vi "CelulaDessalinizadora.vi"() -> ()   [LabVIEW 2014]
panel:
  in  "Adsorção":bool
  in  "OK Button":bool
  in  "Documento de Texto":path
  out "Tempo":dbl
  in  "Condutividade Máxima":dbl
  in  "NÚMERO DE CICLOS":dbl
  in  "Liga/Desliga":bool
  in  "Escolha: Porta Serial":refnum<visa-resource-name>="COM3"
  out "Dessorção":bool
  out "Adsorção":bool
  out "Single-Pass":bool
  out "Batch":bool
  in  "BATCH / SINGLE PASS":bool
  out "Potencial de Célula [mV]":dbl(graph)
  out "pH":dbl(graph)
  out "Condutividade [us/cm]":dbl(graph)
  in  "Selecionar caso":T1(tab)
  in  "TEMPO DE ADSOR敲O P":dbl
  in  "CONDUTIVIDADE \nMÍNIMA NA ADSORÇÃO P":dbl
  in  "TEMPO DE DESSOR敲O P":dbl
  in  "CONDUTIVIDADE \nMÁXIMA NA DESSORÇÃO P":dbl
  in  "Selecionar parâmetro G":enum32{"Tempo", "Condutividade", "Potencial"}(tab)
  in  "TEMPO DE ADSOR敲O G":dbl
  in  "TEMPO DE DESSOR敲O G":dbl
  in  "CONDUTIVIDADE \nMÍNIMA NA ADSORÇÃO G":dbl
  in  "CONDUTIVIDADE \nMÁXIMA NA DESSORÇÃO G":dbl
  in  "POTENCIAL DE CORTE\nNA ADSOR敲O":dbl
  in  "POTENCIAL DE CORTE\nNA DESSOR敲O":dbl
  in  "POTENCIAL DE CORTE\nNA DESSOR敲O G":dbl
  in  "CONDUTIVIDADE \nMÁXIMA NA DESSORÇÃO G2":dbl
  in  "TEMPO DE DESSOR敲O G 2":dbl
  in  "TEMPO DE ADSOR敲O G 2":dbl
  in  "CONDUTIVIDADE \nMÍNIMA NA ADSORÇÃO G 2":dbl
  in  "POTENCIAL DE CORTE\nNA ADSOR敲O G":dbl
  # "CONDUTIVIDADE MÁXIMA"
  # "s"
  # "us/cm"
  # "s"
  # "us/cm"
  # "s"
  # "s"
  # "us/cm"
  # "us/cm"
  # "VV"
  # "V"
  # "s"
  # "us/cm"
  # "mV"
  # "s"
  # "us/cm"
  # "mV"
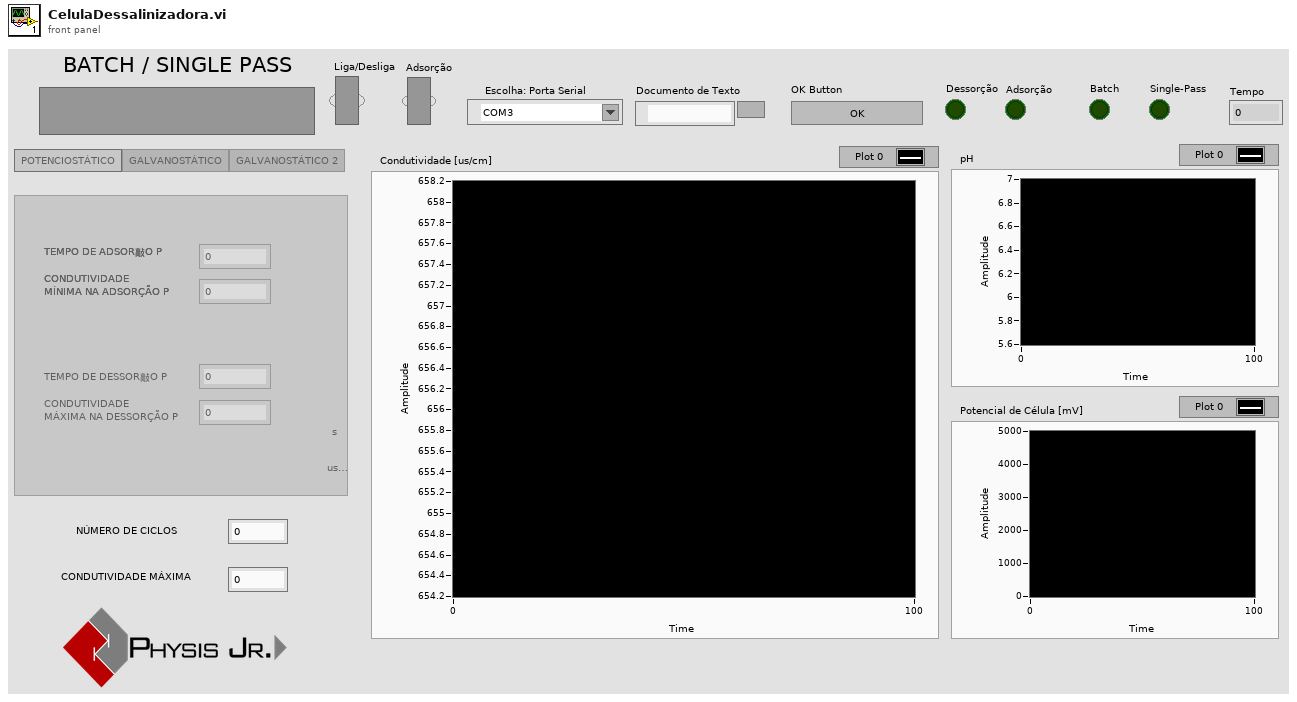
[diagram p1: front panel]
types:
  T1 = enum32{"POTENCIOSTÁTICO", "GALVANOSTÁTICO", "GALVANOSTÁTICO 2"}
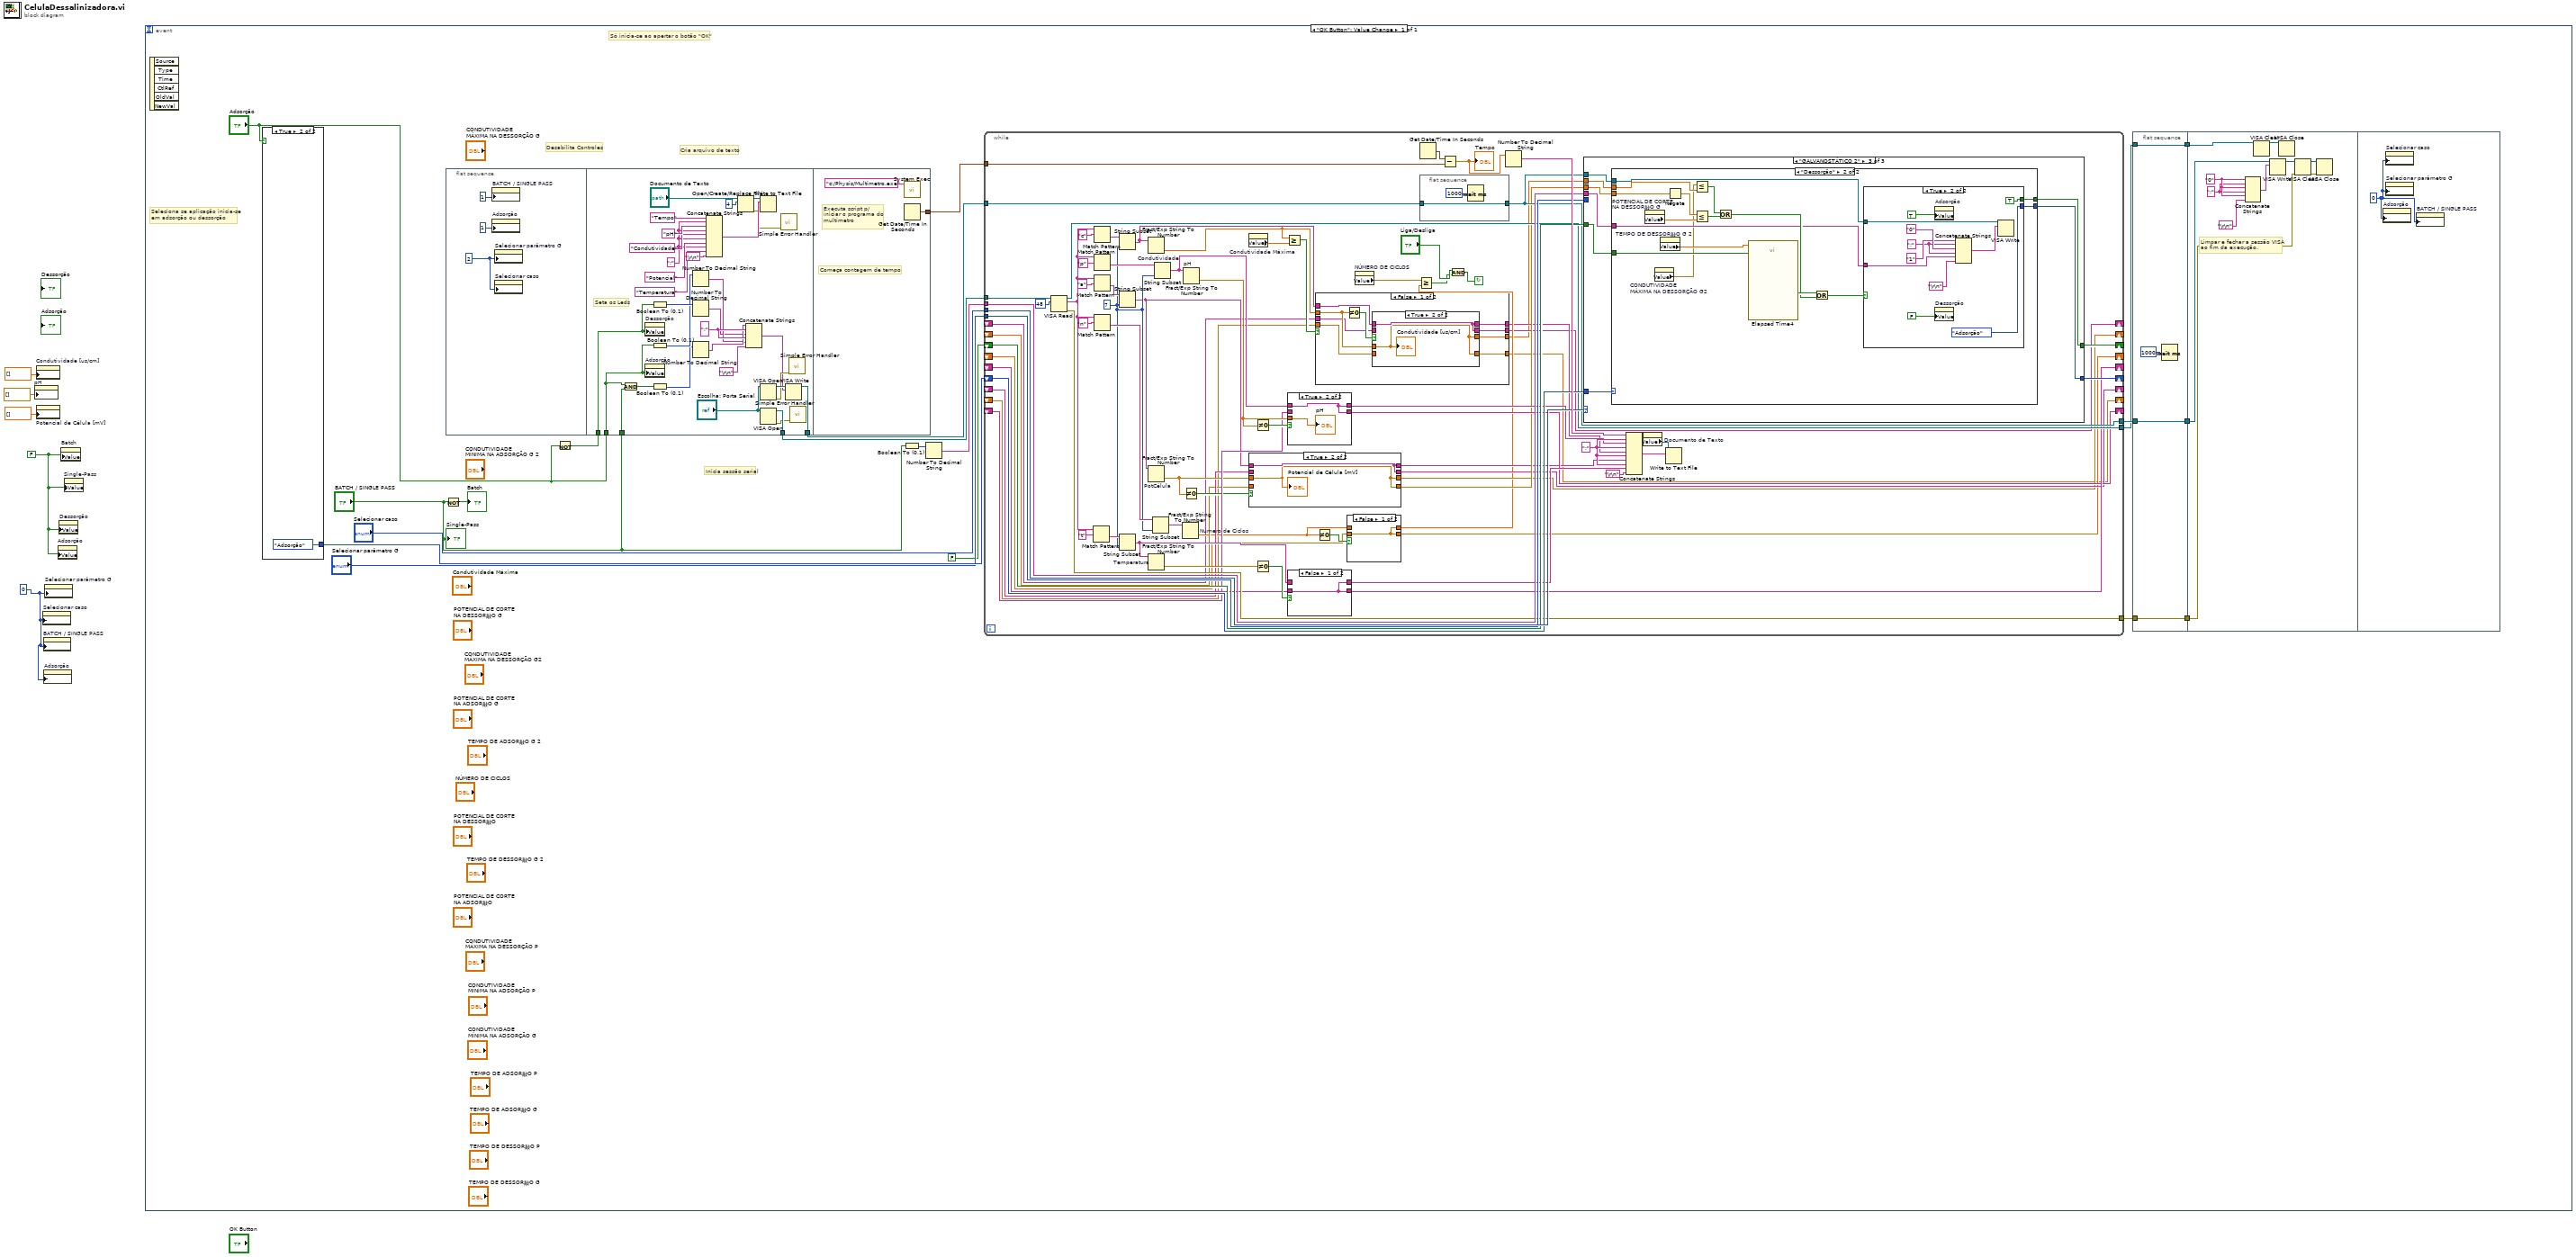
[diagram p0: block diagram]
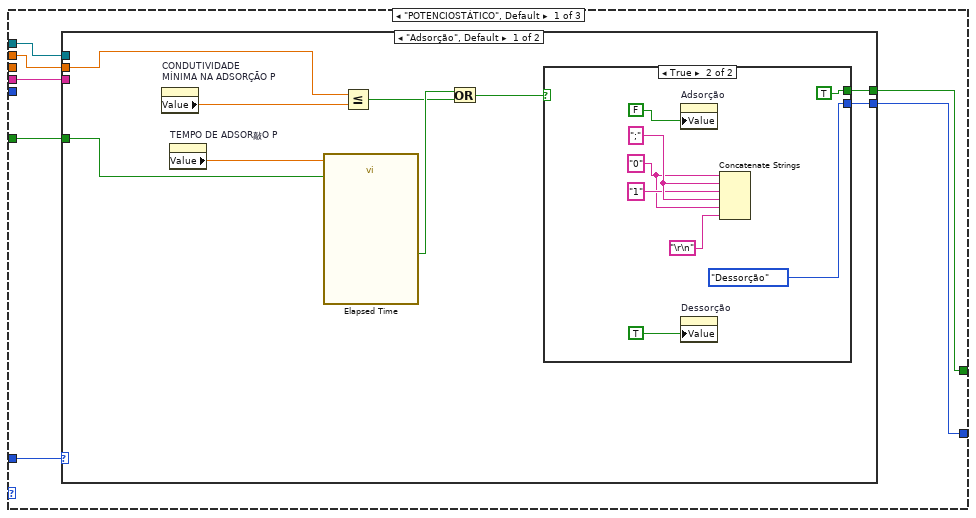
[diagram p6: hidden frame]
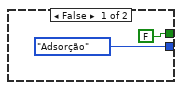
[diagram p7: hidden frame]
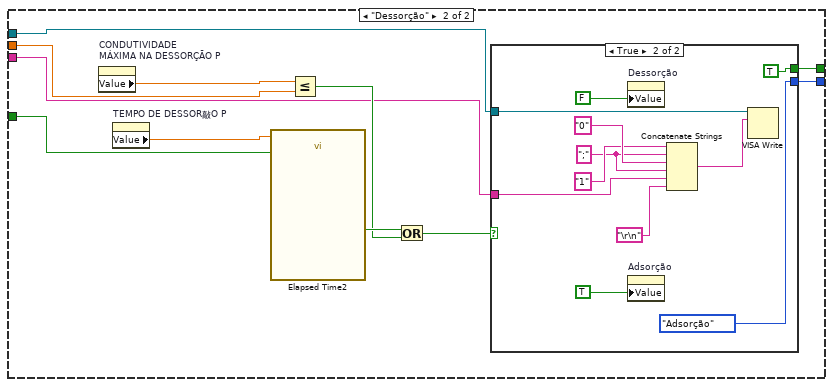
[diagram p8: hidden frame]
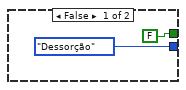
[diagram p9: hidden frame]
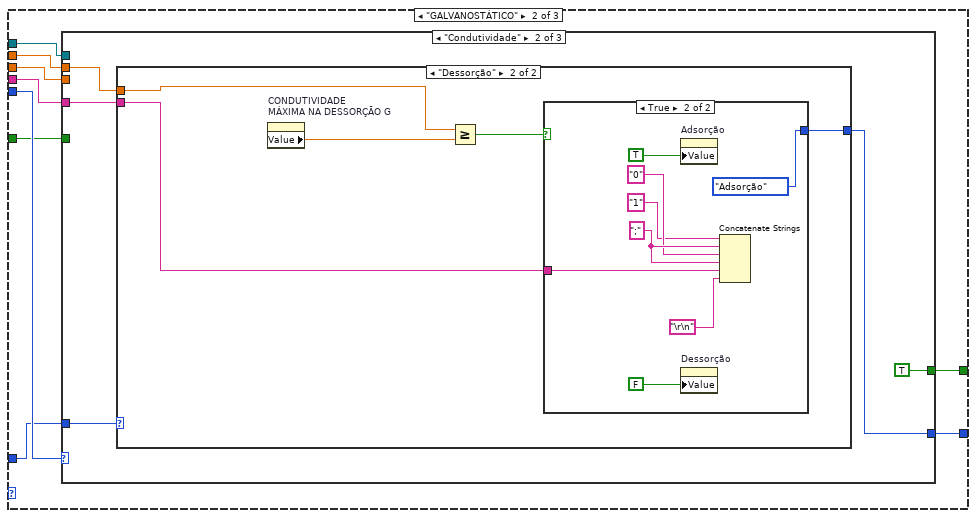
[diagram p10: hidden frame]
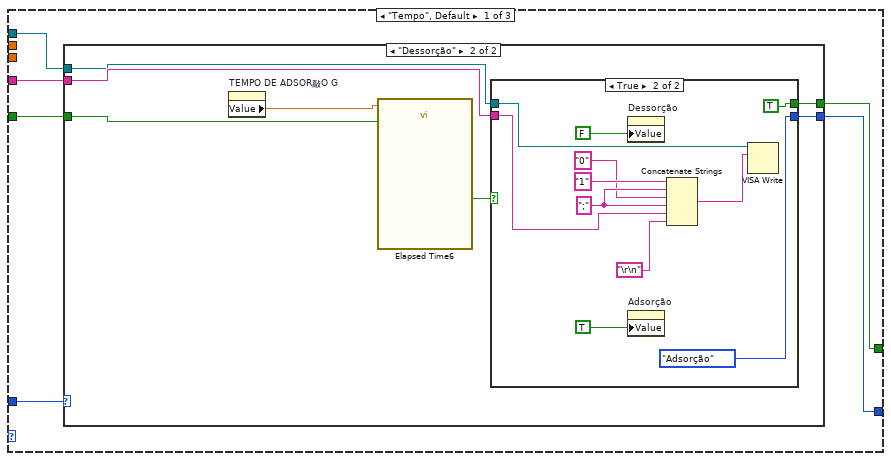
[diagram p11: hidden frame]
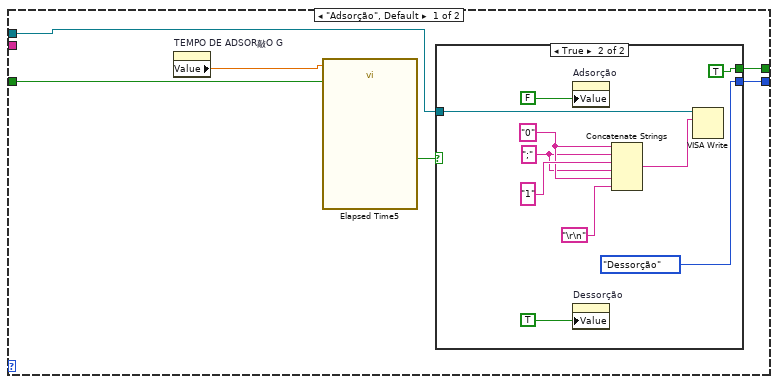
[diagram p12: hidden frame]
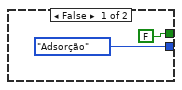
[diagram p13: hidden frame]
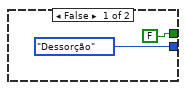
[diagram p14: hidden frame]
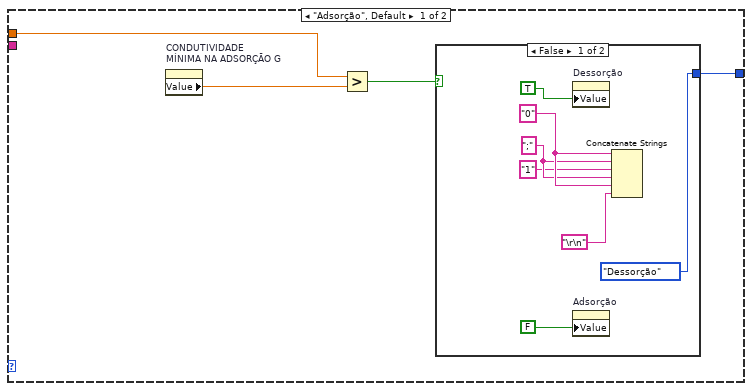
[diagram p15: hidden frame]
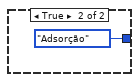
[diagram p16: hidden frame]
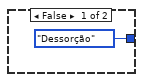
[diagram p17: hidden frame]
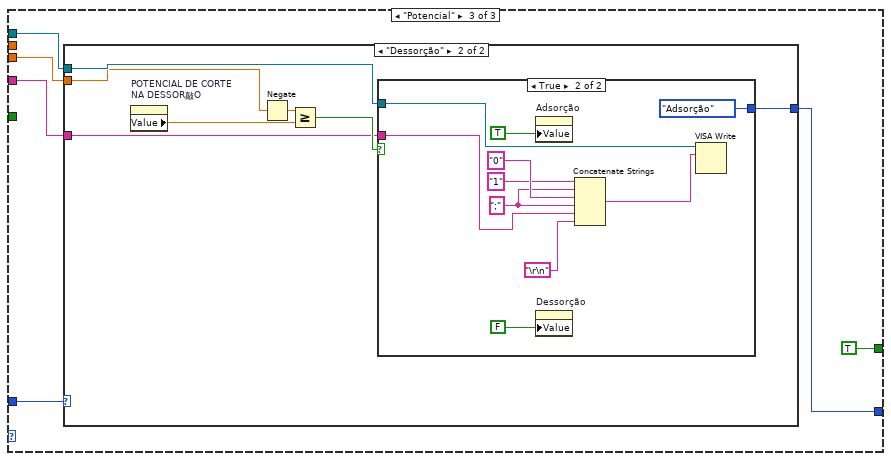
[diagram p18: hidden frame]
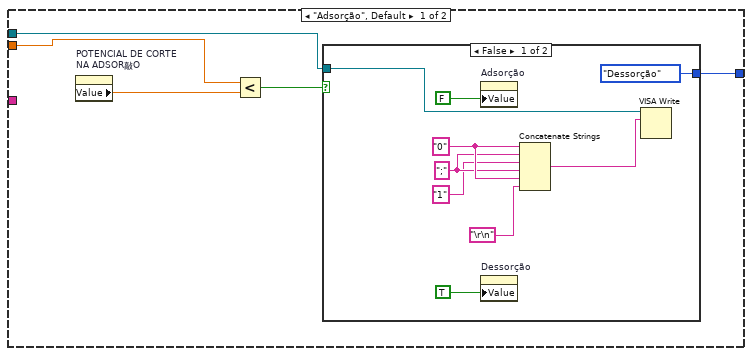
[diagram p19: hidden frame]
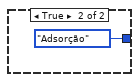
[diagram p20: hidden frame]
diagram:
  w1 = 0
  w2 = FALSE
  n1 = property on="pH" class="WFChart (strict)"("History Data"=dbl[] []) -> ()  [unwired: 2 in, 2 out]
  n2 = property on="Condutividade [us/cm]" class="WFChart (strict)"("History Data"=dbl[] []) -> ()  [unwired: 2 in, 2 out]
  n3 = property on="Potencial de Célula [mV]" class="WFChart (strict)"("History Data"=dbl[] []) -> ()  [unwired: 2 in, 2 out]
  n4 = property on="Selecionar caso" class="TabCtl (strict)"("DisabledEnum"=w1) -> ()  [unwired: 2 in, 2 out]
  n5 = property on="BATCH / SINGLE PASS" class="Bool (strict)"("DisabledEnum"=w1) -> ()  [unwired: 2 in, 2 out]
  n6 = property on="Adsorção" class="Bool (strict)"("DisabledEnum"=w1) -> ()  [unwired: 2 in, 2 out]
  n7 = property on="Selecionar parâmetro G" class="TabCtl (strict)"("DisabledEnum"=w1) -> ()  [unwired: 2 in, 2 out]
  n8 = property on="Adsorção" class="Bool (strict)"("Value"=w2) -> ()  [unwired: 2 in, 2 out]
  n9 = property on="Dessorção" class="Bool (strict)"("Value"=w2) -> ()  [unwired: 2 in, 2 out]
  n10 = property on="Batch" class="Bool (strict)"("Value"=w2) -> ()  [unwired: 2 in, 2 out]
  n11 = property on="Single-Pass" class="Bool (strict)"("Value"=w2) -> ()  [unwired: 2 in, 2 out]
  n12 = event shown="[0] \"OK Button\": Value Change" {
    selector: _ -> [_]
    dyn-events: _ -> [_]
    timeout: _ -> [_]
    event "OK Button": Value Change {
      # "Inicia sessão serial"
      # "Cria arquivo de texto"
      # "Desabilita Controles"
      # "Só inicia-se ao apertar o botão \"OK\""
      # "Seleciona se aplicação inicia-se\nem adsorção ou dessorção"
      n13 = event-data() -> ()  [unwired: 1 in, 6 out]
      n14 = case shown="True" "Adsorção" {
        tunnel: [enum16{"Adsorção", "Dessorção"}."Dessorção" enum16{"Adsorção", "Dessorção"}."Adsorção"] -> w18
        frame False {
        }
        frame True {
        }
      }
      n15 = Not(x="BATCH / SINGLE PASS") -> (.not. x?=→"Batch":bool)
      n16 = flat-sequence {
        tunnel: "Adsorção" -> [w46]
        tunnel: w16 -> [w55]
        tunnel: "BATCH / SINGLE PASS" -> [w58]
        tunnel: [w54] -> w11
        tunnel: [w53] -> w10
        tunnel: [w76] -> w15
        frame #0 {
          w41 = 2
          n17 = property on="BATCH / SINGLE PASS" class="Bool (strict)"("DisabledEnum"=1) -> ()  [unwired: 2 in, 2 out]
          n18 = property on="Adsorção" class="Bool (strict)"("DisabledEnum"=1) -> ()  [unwired: 2 in, 2 out]
          n19 = property on="Selecionar parâmetro G" class="TabCtl (strict)"("DisabledEnum"=w41) -> ()  [unwired: 2 in, 2 out]
          n20 = property on="Selecionar caso" class="TabCtl (strict)"("DisabledEnum"=w41) -> ()  [unwired: 2 in, 2 out]
        }
        frame #1 {
          w62 = ";"
          w66 = ";"
          # "Seta os Leds"
          n21 = And(x=w46, y=w58) -> (x .and. y?=w57:bool)
          n22 = property on="Dessorção" class="Bool (strict)"("Value"=w55) -> ()  [unwired: 2 in, 2 out]
          n23 = property on="Adsorção" class="Bool (strict)"("Value"=w46) -> ()  [unwired: 2 in, 2 out]
          n24 = Boolean To (0,1)(Boolean=w55) -> (0, 1=w60:i16)
          n25 = Boolean To (0,1)(Boolean=w46) -> (0, 1=w59:i16)
          n26 = Boolean To (0,1)(Boolean=w57) -> (0, 1=w56:i16)
          n27 = Number To Decimal String(number=w59) -> (decimal integer string=w48:string)  [unwired: 1 in]
          n28 = Number To Decimal String(number=w60) -> (decimal integer string=w47:string)  [unwired: 1 in]
          n29 = Number To Decimal String(number=w56) -> (decimal integer string=w49:string)  [unwired: 1 in]
          n30 = Concatenate Strings("Tempo", w66, "pH", w66, "Condutividade", w66, "Potencial", w66, "Temperatura", "\r\n") -> (w64:string)
          n31 = Open/Create/Replace File(file path (use dialog)="Documento de Texto", operation (0:open)=4) -> (refnum out=w72:refnum<file>, error out=w52:errorcluster)  [unwired: 4 in, 1 out]
          n32 = Concatenate Strings(w49, w62, w47, w62, w48, "\r\n") -> (w45:string)
          n33 = Write to Text File(file (use dialog)=w72, text=w64) -> ()  [unwired: 2 in, 3 out]
          n34 = VISA Open(VISA resource name="Escolha: Porta Serial") -> (VISA resource name=w61:refnum<visa-resource-name>, error out=w51:errorcluster)  [unwired: 4 in]
          n35 = VISA Open(VISA resource name="Escolha: Porta Serial") -> (VISA resource name=w54:refnum<visa-resource-name>, error out=w50:errorcluster)  [unwired: 4 in]
          n36 = call <vilib>:"Simple Error Handler.vi"("error in (no error)"=w52) -> ()  [unwired: 4 in, 5 out]
          n37 = VISA Write(VISA resource name=w61, write buffer=w45) -> (VISA resource name out=w53:refnum<visa-resource-name>)  [unwired: 1 in, 2 out]
          n38 = call <vilib>:"Simple Error Handler.vi"("error in (no error)"=w51) -> ()  [unwired: 4 in, 5 out]
          n39 = call <vilib>:"Simple Error Handler.vi"("error in (no error)"=w50) -> ()  [unwired: 4 in, 5 out]
        }
        frame #2 {
          # "Executa script p/\niniciar o programa do\nmultímetro"
          # "Começa contagem de tempo"
          n40 = call <vilib>:"System Exec.vi"("command line"="c:/Physis/Multimetro.exe") -> ()  [unwired: 7 in, 4 out]
          n41 = Get Date/Time In Seconds() -> (seconds since 1Jan1904=w76:timestamp)
        }
      }
      n42 = Not(x="Adsorção") -> (.not. x?=w16:bool)
      n43 = Boolean To (0,1)(Boolean="BATCH / SINGLE PASS") -> (0, 1=w13:i16)
      n44 = Number To Decimal String(number=w13) -> (decimal integer string=w12:string)  [unwired: 1 in]
      n45 = while {
        tunnel: w11 -> [w149]
        tunnel: w15 -> [w127]
        tunnel: "Selecionar caso" -> [w126]
        shift-right: [w125] -> _
        shift-left: w18 -> [w124]
        shift-right: [w123] -> _
        shift-left: FALSE -> [w122]
        tunnel: w12 -> [w121]
        tunnel: w10 -> [w119]
        tunnel: "Selecionar parâmetro G" -> [w120]
        tunnel: [w118] -> w9
        tunnel: [w117] -> w8
        tunnel: [w116] -> w7
        shift-right: [w109] -> _
        shift-left: _ -> [w108]
        shift-right: [w103] -> _
        shift-left: _ -> [w102]
        shift-right: [w96] -> _
        shift-left: _ -> [w95]
        shift-right: [w94] -> _
        shift-left: _ -> [w93]
        shift-right: [w89] -> _
        shift-left: _ -> [w88]
        shift-right: [w85] -> _
        shift-left: _ -> [w84]
        shift-right: [w82] -> _
        shift-left: _ -> [w81]
        stop <- w77 continue-if-true
        w131 = ";"
        w138 = 7
        n46 = VISA Read(VISA resource name=w149, byte count=48) -> (VISA resource name out=w117:refnum<visa-resource-name>, read buffer=w136:string, error out=w116:errorcluster)  [unwired: 1 in, 1 out]
        n47 = Match Pattern(string=w136, regular expression="t") -> (after substring=w144:string)  [unwired: 1 in, 3 out]
        n48 = Match Pattern(string=w136, regular expression="c") -> (after substring=w139:string)  [unwired: 1 in, 3 out]
        n49 = Match Pattern(string=w136, regular expression="a") -> (after substring=w142:string)  [unwired: 1 in, 3 out]
        n50 = Match Pattern(string=w136, regular expression="p") -> (after substring=w143:string)  [unwired: 1 in, 3 out]
        n51 = Match Pattern(string=w136, regular expression="n") -> (after substring=w141:string)  [unwired: 1 in, 3 out]
        n52 = String Subset(string=w139, length (rest)=w138) -> (substring=w128:string)  [unwired: 1 in]
        n53 = String Subset(string=w142, length (rest)=w138) -> (substring=w98:string)  [unwired: 1 in]
        n54 = String Subset(string=w144, length (rest)=w138) -> (substring=w111:string)  [unwired: 1 in]
        n55 = Fract/Exp String To Number "Condutividade"(string=w128) -> (number=w87:dbl)  [unwired: 3 in, 1 out]
        n56 = Fract/Exp String To Number "PotCélula"(string=w98) -> (number=w100:dbl)  [unwired: 3 in, 1 out]
        n57 = Fract/Exp String To Number "Temperatura"(string=w111) -> (number=w113:dbl)  [unwired: 3 in, 1 out]
        n58 = String Subset(string=w141, length (rest)=w138) -> (substring=w137:string)  [unwired: 1 in]
        n59 = String Subset(string=w143, length (rest)=w138) -> (substring=w105:string)  [unwired: 1 in]
        n60 = Fract/Exp String To Number "Número de Ciclos"(string=w137) -> (number=w91:dbl)  [unwired: 3 in, 1 out]
        n61 = Fract/Exp String To Number "pH"(string=w105) -> (number=w106:dbl)  [unwired: 3 in, 1 out]
        n62 = Not Equal To 0?(x=w100) -> (x != 0?=w101:bool)
        n63 = property on="Condutividade Máxima" class="DigNum (strict)"() -> ("Value"=w115:dbl)  [unwired: 2 in, 2 out]
        n64 = case shown="True" w101 {
          tunnel: w100 -> [_ w155]
          tunnel: [w153 w155] -> w99
          tunnel: w98 -> [_ w156]
          tunnel: [w154 w156] -> w97
          tunnel: [w154 w156] -> w96
          tunnel: w95 -> [w154 _]
          tunnel: [w153 w155] -> w94
          tunnel: w93 -> [w153 _]
          frame False {
          }
          frame True {
            "Potencial de Célula [mV]" <- w155
          }
        }
        n65 = Not Equal To 0?(x=w106) -> (x != 0?=w107:bool)
        n66 = Not Equal To 0?(x=w113) -> (x != 0?=w112:bool)
        n67 = Greater Or Equal?(x=w87, y=w115) -> (x >= y?=w129:bool)
        n68 = case shown="True" w107 {
          tunnel: w106 -> [_ w159]
          tunnel: w105 -> [_ w158]
          tunnel: [w157 w158] -> w104
          tunnel: [w157 w158] -> w103
          tunnel: w102 -> [w157 _]
          frame False {
          }
          frame True {
            "pH" <- w159
          }
        }
        n69 = case shown="False" w112 {
          tunnel: w111 -> [_ w161]
          tunnel: [w160 w161] -> w110
          tunnel: [w160 w161] -> w109
          tunnel: w108 -> [w160 _]
          frame False {
          }
          frame True {
          }
        }
        n70 = case shown="False" w129 {
          tunnel: w128 -> [w405 _]
          tunnel: w87 -> [w407 _]
          tunnel: [w406 w414] -> w86
          tunnel: [w404 w414] -> w85
          tunnel: w84 -> [w403 w414]
          tunnel: [w402 w413] -> w83
          tunnel: [w401 w413] -> w82
          tunnel: w81 -> [w400 w413]
          frame False {
            n71 = Not Equal To 0?(x=w407) -> (x != 0?=w408:bool)
            n72 = case shown="True" w408 {
              tunnel: w407 -> [_ w411]
              tunnel: [w410 w412] -> w406
              tunnel: w405 -> [_ w412]
              tunnel: [w410 w412] -> w404
              tunnel: w403 -> [w410 _]
              tunnel: [w409 w411] -> w402
              tunnel: [w409 w411] -> w401
              tunnel: w400 -> [w409 _]
              frame False {
              }
              frame True {
                "Condutividade [us/cm]" <- w411
              }
            }
          }
          frame True {
          }
        }
        n73 = Not Equal To 0?(x=w91) -> (x != 0?=w92:bool)
        n74 = case shown="False" w92 {
          tunnel: w91 -> [_ w152]
          tunnel: [w151 w152] -> w90
          tunnel: [w151 w152] -> w89
          tunnel: w88 -> [w151 _]
          frame False {
          }
          frame True {
          }
        }
        n75 = property on="NÚMERO DE CICLOS" class="DigNum (strict)"() -> ("Value"=w114:dbl)  [unwired: 2 in, 2 out]
        n76 = Greater Or Equal?(x=w114, y=w90) -> (x >= y?=w78:bool)
        n77 = Get Date/Time In Seconds() -> (seconds since 1Jan1904=w135:timestamp)
        n78 = flat-sequence {
          tunnel: [w162] -> w118
          tunnel: w119 -> [w162]
          frame #0 {
            n79 = Wait (ms)(milliseconds to wait=1000) -> ()  [unwired: 1 out]
          }
        }
        n80 = Subtract(x=w135, y=w127) -> (x-y=w134:dbl)
        "Tempo" <- w134
        n81 = And(x="Liga/Desliga", y=w78) -> (x .and. y?=w77:bool)
        n82 = Number To Decimal String(number=w134) -> (decimal integer string=w132:string)  [unwired: 1 in]
        n83 = case shown="\"GALVANOSTÁTICO 2\"" w126 {
          tunnel: w83 -> [w164 w215 w342]
          tunnel: [w170 w219 w340] -> w125
          tunnel: w124 -> [w167 w221 w344]
          tunnel: [w169 w218 w339] -> w123
          tunnel: w122 -> [w168 w220 w343]
          tunnel: w121 -> [w166 w216 w337]
          tunnel: w99 -> [_ w214 w341]
          tunnel: w118 -> [w165 w217 w338]
          tunnel: w120 -> [_ w222 _]
          frame "POTENCIOSTÁTICO", Default {
            n84 = case shown="\"Adsorção\", Default" w167 {
              tunnel: w164 -> [w179 w199]
              tunnel: [w175 w195] -> w170
              tunnel: [w174 w194] -> w169
              tunnel: w168 -> [w173 w200]
              tunnel: w166 -> [_ w193]
              tunnel: w165 -> [_ w192]
              frame "Adsorção", Default {
                n85 = property on="CONDUTIVIDADE \nMÍNIMA NA ADSORÇÃO P" class="DigNum (strict)"() -> ("Value"=w172:dbl)  [unwired: 2 in, 2 out]
                n86 = property on="TEMPO DE ADSOR敲O P" class="DigNum (strict)"() -> ("Value"=w171:dbl)  [unwired: 2 in, 2 out]
                n87 = call "Elapsed Time"("Time Target (s)"=w171, "Reset"=w173) -> ("Time has Elapsed"=w178:bool)  [unwired: 10 in, 7 out]
                n88 = Less Or Equal?(x=w179, y=w172) -> (x <= y?=w177:bool)
                n89 = Or(x=w178, y=w177) -> (x .or. y?=w176:bool)
                n90 = case shown="True" w176 {
                  tunnel: [enum16{"Adsorção", "Dessorção"}."Adsorção" enum16{"Adsorção", "Dessorção"}."Dessorção"] -> w175
                  tunnel: [FALSE TRUE] -> w174
                  frame False {
                  }
                  frame True {
                    w182 = "0"
                    w185 = ";"
                    n91 = property on="Adsorção" class="Bool (strict)"("Value"=FALSE) -> ()  [unwired: 2 in, 2 out]
                    n92 = property on="Dessorção" class="Bool (strict)"("Value"=TRUE) -> ()  [unwired: 2 in, 2 out]
                    n93 = Concatenate Strings(w182, w185, "1", w185, w182, "\r\n") -> ()  [unwired: 1 out]
                  }
                }
              }
              frame "Dessorção" {
                n94 = property on="CONDUTIVIDADE \nMÁXIMA NA DESSORÇÃO P" class="DigNum (strict)"() -> ("Value"=w190:dbl)  [unwired: 2 in, 2 out]
                n95 = property on="TEMPO DE DESSOR敲O P" class="DigNum (strict)"() -> ("Value"=w191:dbl)  [unwired: 2 in, 2 out]
                n96 = call "Elapsed Time2"("Time Target (s)"=w191, "Reset"=w200) -> ("Time has Elapsed"=w198:bool)  [unwired: 10 in, 7 out]
                n97 = Less Or Equal?(x=w190, y=w199) -> (x <= y?=w197:bool)
                n98 = Or(x=w198, y=w197) -> (x .or. y?=w196:bool)
                n99 = case shown="True" w196 {
                  tunnel: [enum16{"Adsorção", "Dessorção"}."Dessorção" enum16{"Adsorção", "Dessorção"}."Adsorção"] -> w195
                  tunnel: [FALSE TRUE] -> w194
                  tunnel: w193 -> [_ w208]
                  tunnel: w192 -> [_ w206]
                  frame False {
                  }
                  frame True {
                    w204 = ";"
                    n100 = property on="Dessorção" class="Bool (strict)"("Value"=FALSE) -> ()  [unwired: 2 in, 2 out]
                    n101 = property on="Adsorção" class="Bool (strict)"("Value"=TRUE) -> ()  [unwired: 2 in, 2 out]
                    n102 = Concatenate Strings("1", w204, "0", w204, w208, "\r\n") -> (w205:string)
                    n103 = VISA Write(VISA resource name=w206, write buffer=w205) -> ()  [unwired: 1 in, 3 out]
                  }
                }
              }
            }
          }
          frame "GALVANOSTÁTICO" {
            n104 = case shown="\"Condutividade\"" w222 {
              tunnel: w221 -> [w228 w271 w302]
              tunnel: w220 -> [w227 _ _]
              tunnel: [w226 w269 w300] -> w219
              tunnel: [w225 TRUE TRUE] -> w218
              tunnel: w217 -> [w224 _ w299]
              tunnel: w216 -> [w223 w267 w298]
              tunnel: w215 -> [_ w270 _]
              tunnel: w214 -> [_ _ w301]
              frame "Tempo", Default {
                n105 = case shown="\"Dessorção\"" w228 {
                  tunnel: w227 -> [w234 w253]
                  tunnel: [w232 w251] -> w226
                  tunnel: [w231 w250] -> w225
                  tunnel: w224 -> [w230 w248]
                  tunnel: w223 -> [_ w249]
                  frame "Adsorção", Default {
                    n106 = property on="TEMPO DE ADSOR敲O G" class="DigNum (strict)"() -> ("Value"=w229:dbl)  [unwired: 2 in, 2 out]
                    n107 = call "Elapsed Time5"("Time Target (s)"=w229, "Reset"=w234) -> ("Time has Elapsed"=w233:bool)  [unwired: 10 in, 7 out]
                    n108 = case shown="True" w233 {
                      tunnel: [enum16{"Adsorção", "Dessorção"}."Adsorção" enum16{"Adsorção", "Dessorção"}."Dessorção"] -> w232
                      tunnel: [FALSE TRUE] -> w231
                      tunnel: w230 -> [_ w239]
                      frame False {
                      }
                      frame True {
                        w241 = "0"
                        w238 = ";"
                        n109 = property on="Adsorção" class="Bool (strict)"("Value"=FALSE) -> ()  [unwired: 2 in, 2 out]
                        n110 = property on="Dessorção" class="Bool (strict)"("Value"=TRUE) -> ()  [unwired: 2 in, 2 out]
                        n111 = Concatenate Strings(w241, w238, "1", w238, w241, "\r\n") -> (w240:string)
                        n112 = VISA Write(VISA resource name=w239, write buffer=w240) -> ()  [unwired: 1 in, 3 out]
                      }
                    }
                  }
                  frame "Dessorção" {
                    n113 = property on="TEMPO DE ADSOR敲O G" class="DigNum (strict)"() -> ("Value"=w247:dbl)  [unwired: 2 in, 2 out]
                    n114 = call "Elapsed Time6"("Time Target (s)"=w247, "Reset"=w253) -> ("Time has Elapsed"=w252:bool)  [unwired: 10 in, 7 out]
                    n115 = case shown="True" w252 {
                      tunnel: [enum16{"Adsorção", "Dessorção"}."Dessorção" enum16{"Adsorção", "Dessorção"}."Adsorção"] -> w251
                      tunnel: [FALSE TRUE] -> w250
                      tunnel: w249 -> [_ w259]
                      tunnel: w248 -> [_ w257]
                      frame False {
                      }
                      frame True {
                        w262 = ";"
                        n116 = property on="Dessorção" class="Bool (strict)"("Value"=FALSE) -> ()  [unwired: 2 in, 2 out]
                        n117 = property on="Adsorção" class="Bool (strict)"("Value"=TRUE) -> ()  [unwired: 2 in, 2 out]
                        n118 = Concatenate Strings("1", w262, "0", w262, w259, "\r\n") -> (w258:string)
                        n119 = VISA Write(VISA resource name=w257, write buffer=w258) -> ()  [unwired: 1 in, 3 out]
                      }
                    }
                  }
                }
              }
              frame "Condutividade" {
                n120 = case shown="\"Dessorção\"" w271 {
                  tunnel: w270 -> [w275 w288]
                  tunnel: [w273 w286] -> w269
                  tunnel: w267 -> [_ w285]
                  frame "Adsorção", Default {
                    n121 = property on="CONDUTIVIDADE \nMÍNIMA NA ADSORÇÃO G" class="DigNum (strict)"() -> ("Value"=w272:dbl)  [unwired: 2 in, 2 out]
                    n122 = Greater?(x=w275, y=w272) -> (0:w274:bool)
                    n123 = case shown="False" w274 {
                      tunnel: [enum16{"Adsorção", "Dessorção"}."Dessorção" enum16{"Adsorção", "Dessorção"}."Adsorção"] -> w273
                      frame False {
                        w279 = "0"
                        w278 = ";"
                        n124 = property on="Dessorção" class="Bool (strict)"("Value"=TRUE) -> ()  [unwired: 2 in, 2 out]
                        n125 = property on="Adsorção" class="Bool (strict)"("Value"=FALSE) -> ()  [unwired: 2 in, 2 out]
                        n126 = Concatenate Strings(w279, w278, "1", w278, w279, "\r\n") -> ()  [unwired: 1 out]
                      }
                      frame True {
                      }
                    }
                  }
                  frame "Dessorção" {
                    n127 = property on="CONDUTIVIDADE \nMÁXIMA NA DESSORÇÃO G" class="DigNum (strict)"() -> ("Value"=w284:dbl)  [unwired: 2 in, 2 out]
                    n128 = Greater Or Equal?(x=w288, y=w284) -> (x >= y?=w287:bool)
                    n129 = case shown="True" w287 {
                      tunnel: [enum16{"Adsorção", "Dessorção"}."Dessorção" enum16{"Adsorção", "Dessorção"}."Adsorção"] -> w286
                      tunnel: w285 -> [_ w293]
                      frame False {
                      }
                      frame True {
                        w294 = ";"
                        n130 = property on="Adsorção" class="Bool (strict)"("Value"=TRUE) -> ()  [unwired: 2 in, 2 out]
                        n131 = property on="Dessorção" class="Bool (strict)"("Value"=FALSE) -> ()  [unwired: 2 in, 2 out]
                        n132 = Concatenate Strings("1", w294, "0", w294, w293, "\r\n") -> ()  [unwired: 1 out]
                      }
                    }
                  }
                }
              }
              frame "Potencial" {
                n133 = case shown="\"Dessorção\"" w302 {
                  tunnel: w301 -> [w304 w319]
                  tunnel: [w307 w324] -> w300
                  tunnel: w299 -> [w306 w322]
                  tunnel: w298 -> [_ w323]
                  frame "Adsorção", Default {
                    n134 = property on="POTENCIAL DE CORTE\nNA ADSOR敲O" class="DigNum (strict)"() -> ("Value"=w305:dbl)  [unwired: 2 in, 2 out]
                    n135 = Less?(x=w304, y=w305) -> (x < y?=w308:bool)
                    n136 = case shown="False" w308 {
                      tunnel: [enum16{"Adsorção", "Dessorção"}."Dessorção" enum16{"Adsorção", "Dessorção"}."Adsorção"] -> w307
                      tunnel: w306 -> [w315 _]
                      frame False {
                        w312 = "0"
                        w311 = ";"
                        n137 = property on="Adsorção" class="Bool (strict)"("Value"=FALSE) -> ()  [unwired: 2 in, 2 out]
                        n138 = property on="Dessorção" class="Bool (strict)"("Value"=TRUE) -> ()  [unwired: 2 in, 2 out]
                        n139 = Concatenate Strings(w312, w311, "1", w311, w312, "\r\n") -> (w316:string)
                        n140 = VISA Write(VISA resource name=w315, write buffer=w316) -> ()  [unwired: 1 in, 3 out]
                      }
                      frame True {
                      }
                    }
                  }
                  frame "Dessorção" {
                    n141 = property on="POTENCIAL DE CORTE\nNA DESSOR敲O" class="DigNum (strict)"() -> ("Value"=w321:dbl)  [unwired: 2 in, 2 out]
                    n142 = Negate(x=w319) -> (-x=w320:dbl)
                    n143 = Greater Or Equal?(x=w320, y=w321) -> (x >= y?=w325:bool)
                    n144 = case shown="True" w325 {
                      tunnel: [enum16{"Adsorção", "Dessorção"}."Dessorção" enum16{"Adsorção", "Dessorção"}."Adsorção"] -> w324
                      tunnel: w323 -> [_ w332]
                      tunnel: w322 -> [_ w330]
                      frame False {
                      }
                      frame True {
                        w329 = ";"
                        n145 = property on="Adsorção" class="Bool (strict)"("Value"=TRUE) -> ()  [unwired: 2 in, 2 out]
                        n146 = property on="Dessorção" class="Bool (strict)"("Value"=FALSE) -> ()  [unwired: 2 in, 2 out]
                        n147 = Concatenate Strings("1", w329, "0", w329, w332, "\r\n") -> (w331:string)
                        n148 = VISA Write(VISA resource name=w330, write buffer=w331) -> ()  [unwired: 1 in, 3 out]
                      }
                    }
                  }
                }
              }
            }
          }
          frame "GALVANOSTÁTICO 2" {
            n149 = case shown="\"Dessorção\"" w344 {
              tunnel: w343 -> [w358 w386]
              tunnel: w342 -> [w357 w385]
              tunnel: w341 -> [w356 w383]
              tunnel: [w350 w377] -> w340
              tunnel: [w349 w376] -> w339
              tunnel: w338 -> [w348 w375]
              tunnel: w337 -> [_ w374]
              frame "Adsorção", Default {
                n150 = property on="CONDUTIVIDADE \nMÍNIMA NA ADSORÇÃO G 2" class="DigNum (strict)"() -> ("Value"=w347:dbl)  [unwired: 2 in, 2 out]
                n151 = property on="POTENCIAL DE CORTE\nNA ADSOR敲O G" class="DigNum (strict)"() -> ("Value"=w346:dbl)  [unwired: 2 in, 2 out]
                n152 = property on="TEMPO DE ADSOR敲O G 2" class="DigNum (strict)"() -> ("Value"=w345:dbl)  [unwired: 2 in, 2 out]
                n153 = Less Or Equal?(x=w357, y=w347) -> (x <= y?=w355:bool)
                n154 = Less Or Equal?(x=w346, y=w356) -> (x <= y?=w354:bool)
                n155 = Or(x=w355, y=w354) -> (x .or. y?=w352:bool)
                n156 = call "Elapsed Time3"("Time Target (s)"=w345, "Reset"=w358) -> ("Time has Elapsed"=w353:bool)  [unwired: 10 in, 7 out]
                n157 = Or(x=w353, y=w352) -> (x .or. y?=w351:bool)
                n158 = case shown="True" w351 {
                  tunnel: [enum16{"Adsorção", "Dessorção"}."Adsorção" enum16{"Adsorção", "Dessorção"}."Dessorção"] -> w350
                  tunnel: [FALSE TRUE] -> w349
                  tunnel: w348 -> [_ w363]
                  frame False {
                  }
                  frame True {
                    w365 = "0"
                    w362 = ";"
                    n159 = property on="Adsorção" class="Bool (strict)"("Value"=FALSE) -> ()  [unwired: 2 in, 2 out]
                    n160 = property on="Dessorção" class="Bool (strict)"("Value"=TRUE) -> ()  [unwired: 2 in, 2 out]
                    n161 = Concatenate Strings(w365, w362, "1", w362, w365, "\r\n") -> (w364:string)
                    n162 = VISA Write(VISA resource name=w363, write buffer=w364) -> ()  [unwired: 1 in, 3 out]
                  }
                }
              }
              frame "Dessorção" {
                n163 = property on="POTENCIAL DE CORTE\nNA DESSOR敲O G" class="DigNum (strict)"() -> ("Value"=w372:dbl)  [unwired: 2 in, 2 out]
                n164 = property on="CONDUTIVIDADE \nMÁXIMA NA DESSORÇÃO G2" class="DigNum (strict)"() -> ("Value"=w371:dbl)  [unwired: 2 in, 2 out]
                n165 = property on="TEMPO DE DESSOR敲O G 2" class="DigNum (strict)"() -> ("Value"=w373:dbl)  [unwired: 2 in, 2 out]
                n166 = Negate(x=w383) -> (-x=w384:dbl)
                n167 = Less Or Equal?(x=w371, y=w385) -> (x <= y?=w382:bool)
                n168 = Less Or Equal?(x=w384, y=w372) -> (x <= y?=w381:bool)
                n169 = Or(x=w382, y=w381) -> (x .or. y?=w379:bool)
                n170 = call "Elapsed Time4"("Time Target (s)"=w373, "Reset"=w386) -> ("Time has Elapsed"=w380:bool)  [unwired: 10 in, 7 out]
                n171 = Or(x=w380, y=w379) -> (x .or. y?=w378:bool)
                n172 = case shown="True" w378 {
                  tunnel: [enum16{"Adsorção", "Dessorção"}."Dessorção" enum16{"Adsorção", "Dessorção"}."Adsorção"] -> w377
                  tunnel: [FALSE TRUE] -> w376
                  tunnel: w375 -> [_ w394]
                  tunnel: w374 -> [_ w391]
                  frame False {
                  }
                  frame True {
                    w390 = ";"
                    n173 = property on="Adsorção" class="Bool (strict)"("Value"=TRUE) -> ()  [unwired: 2 in, 2 out]
                    n174 = property on="Dessorção" class="Bool (strict)"("Value"=FALSE) -> ()  [unwired: 2 in, 2 out]
                    n175 = Concatenate Strings("1", w390, "0", w390, w391, "\r\n") -> (w395:string)
                    n176 = VISA Write(VISA resource name=w394, write buffer=w395) -> ()  [unwired: 1 in, 3 out]
                  }
                }
              }
            }
          }
        }
        n177 = Concatenate Strings(w132, w131, w104, w131, w86, w131, w97, w131, w110, "\r\n") -> (w133:string)
        n178 = property on="Documento de Texto" class="Path"() -> ("Value"=w80:path)  [unwired: 2 in, 2 out]
        n179 = Write to Text File(file (use dialog)=w80, text=w133) -> ()  [unwired: 2 in, 3 out]
      }
      n180 = flat-sequence {
        tunnel: w9 -> [w26]
        tunnel: w7 -> [w27]
        tunnel: w8 -> [w28]
        tunnel: [w28] -> w24
        tunnel: [w27] -> w23
        tunnel: [w26] -> w22
        tunnel: w24 -> [w34]
        tunnel: w23 -> [w33]
        tunnel: w22 -> [w31]
        frame #0 {
          n181 = Wait (ms)(milliseconds to wait=1000) -> ()  [unwired: 1 out]
        }
        frame #1 {
          w32 = "0"
          w30 = ";"
          # "Limpar e fechar a sessão VISA\nao fim da execução."
          n182 = Concatenate Strings(w32, w30, w32, w30, w32, "\r\n") -> (w38:string)
          n183 = VISA Clear(VISA resource name=w34) -> (VISA resource name out=w35:refnum<visa-resource-name>)  [unwired: 1 in, 1 out]
          n184 = VISA Write(VISA resource name=w31, write buffer=w38) -> (VISA resource name out=w39:refnum<visa-resource-name>)  [unwired: 1 in, 2 out]
          n185 = VISA Close(VISA resource name=w35) -> ()  [unwired: 1 in, 1 out]
          n186 = VISA Clear(VISA resource name=w39, error in (no error)=w33) -> (VISA resource name out=w36:refnum<visa-resource-name>, error out=w37:errorcluster)
          n187 = VISA Close(VISA resource name=w36, error in (no error)=w37) -> ()  [unwired: 1 out]
        }
        frame #2 {
          w40 = 0
          n188 = property on="Adsorção" class="Bool (strict)"("DisabledEnum"=w40) -> ()  [unwired: 2 in, 2 out]
          n189 = property on="Selecionar caso" class="TabCtl (strict)"("DisabledEnum"=w40) -> ()  [unwired: 2 in, 2 out]
          n190 = property on="Selecionar parâmetro G" class="TabCtl (strict)"("DisabledEnum"=w40) -> ()  [unwired: 2 in, 2 out]
          n191 = property on="BATCH / SINGLE PASS" class="Bool (strict)"("DisabledEnum"=w40) -> ()  [unwired: 2 in, 2 out]
        }
      }
      "Single-Pass" <- "BATCH / SINGLE PASS"
    }
  }
